vi "Append Rx Map Key to String.vi"(10 "key":T1, 11 "initial string":string) -> (3 "String out":string)   [LabVIEW 2020]
uses:
  Git/niveristand-ballard-milStd1553-custom-device/Source/Custom Device Support/Shared/Message Map Key.ctl
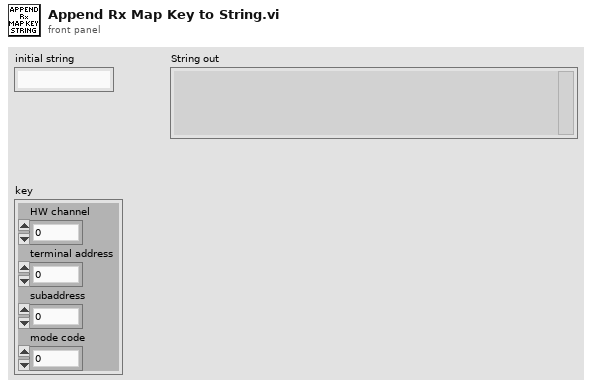
[diagram p1: front panel]
types:
  T1 = typedef "Message Map Key.ctl" = cluster{"HW channel":u16, "terminal address":u16, "subaddress":u16, "mode code":u16}
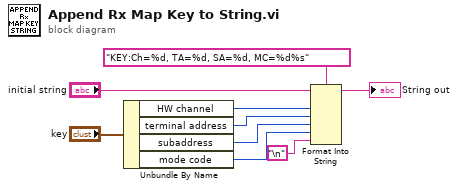
[diagram p0: block diagram]
diagram:
  n1 = Unbundle By Name("key") -> ("HW channel"=w2:u16, "terminal address"=w3:u16, "subaddress"=w4:u16, "mode code"=w5:u16)
  n2 = Format Into String(format string="KEY:Ch=%d, TA=%d, SA=%d, MC=%d%s", initial string="initial string", w2, w3, w4, w5, "\n" ("format string")) -> (resulting string=→"String out":string)  [unwired: 1 in, 1 out]
